vi "WriteCSV.vi"(11 "Log Queue":refnum<queue>) -> (2 "queue out":refnum<queue>, 3 "refnum out":refnum<file>)   [LabVIEW 2026]
uses:
  <vilib>/Platform/TimedLoop/XDataNode/timing_clust.ctl
  <vilib>/Platform/TimedLoop/XDataNode/nitl_modes.ctl
  <vilib>/Platform/TimedLoop/XDataNode/wakeup.ctl
  <vilib>/platform/TimedLoop/XDataNode/XDataNode.xnode
  <vilib>/Platform/TimedLoop/XDataNode/XDNodeRunTimeDep.lvlib
panel:
  in  "datalog":bool
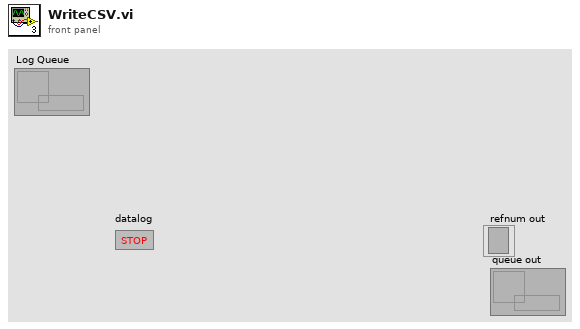
[diagram p1: front panel]
types:
  T1 = enum16{"open", "replace", "create", "open or create", "replace or create", "replace or create with confirmation"}
  T2 = typedef "XDNodeRunTimeDep.lvlib/timing_clust.ctl" = cluster{"Expected End [f-1]":u64, "Actual End [f-1]":u64, "Finished Late? [f-1]":bool, "Expected End [i-1]":u64, "Actual End [i-1]":u64, "Finished Late? [i-1]":bool, "Expected Start [i]":u64, "Actual Start [i]":u64, "Expected Start [f]":u64, "Actual Start [f]":u64, "Source Name":string, "Structure Name":string, "Period":i64, "Deadline":i64, "Offset":i64, "Start":i64, "Priority":i32, "Timeout":i32, "Mode":T3, "Wakeup Reason":T4, "Error":errorcluster, "Source Type":string, "Secondary Source Type":string, "Global End Time":u64, "Global Start Time":u64, "Frame Duration":u64, "Iteration Duration":u64, "Assigned CPU":i32, "I/O Scan Engine Mode":u32}
  T3 = typedef "XDNodeRunTimeDep.lvlib/nitl_modes.ctl" = enum32{"No Change", "Process missed periods, maintain original phase", "Discard missed periods, maintain original phase", "Process missed periods, ignore original phase", "Discard missed periods, ignore original phase"}
  T4 = typedef "XDNodeRunTimeDep.lvlib/wakeup.ctl" = enum32{"Normal", "Aborted", "Asynchronous wakeup", "Timing source error", "Timed loop error", "Timeout"}
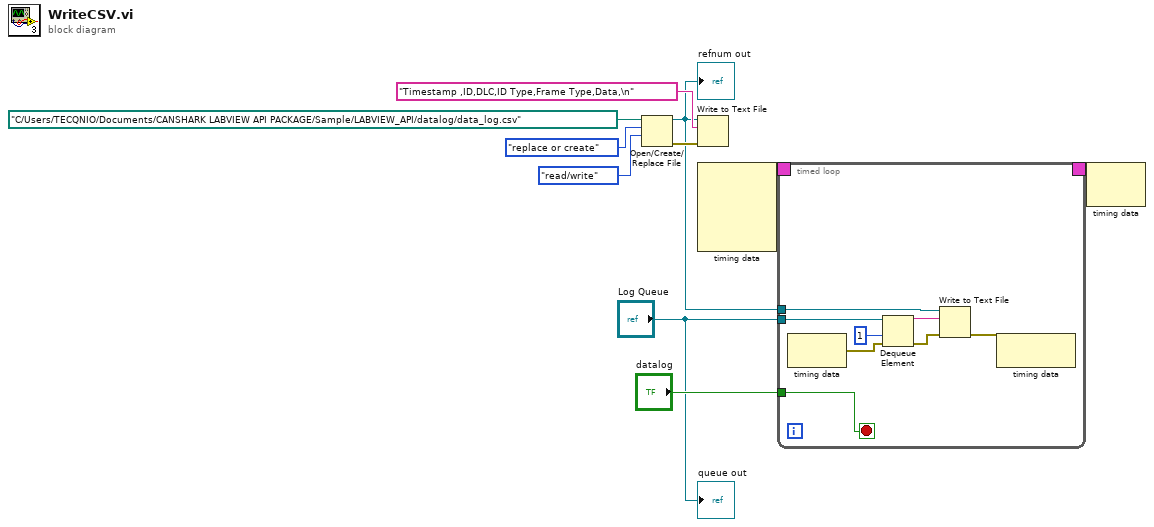
[diagram p0: block diagram]
diagram:
  n1 = Open/Create/Replace File(file path (use dialog)=path "C:/Users/TECQNIO/Documents/CANSHARK LABVIEW API PACKAGE/Sample/LABVIEW_API/datalog/data_log.csv", operation (0:open)=T1."replace or create", access (0:read/write)=enum16{"read/write", "read-only", "write-only"}."read/write") -> (refnum out=w3:refnum<file>, error out=w4:errorcluster)  [unwired: 3 in, 1 out]
  "refnum out" <- w3
  n2 = Write to Text File(file (use dialog)=w3, text="Timestamp ,ID,DLC,ID Type,Frame Type,Data,\n", error in=w4) -> ()  [unwired: 1 in, 3 out]
  n3 = node-c288() -> (w10:T2)  [unwired: 4 in]
  n4 = timed-loop {
    timing: w10 -> [_]
    timing-out: [_] -> w9
    tunnel: "Log Queue" -> [w17]
    tunnel: w3 -> [w15]
    tunnel: "datalog" -> [w14]
    stop <- w14 stop-if-true
    n5 = node-c288() -> (w12:errorcluster)  [unwired: 1 in]
    n6 = Dequeue Element(queue=w17, timeout in ms (-1)=1, error in (no error)=w12) -> (element=w16:string, error out=w11:errorcluster)  [unwired: 2 out]
    n7 = Write to Text File(file (use dialog)=w15, text=w16, error in=w11) -> (error out=w13:errorcluster)  [unwired: 1 in, 2 out]
    n8 = node-c288(w13) -> ()  [unwired: 1 out]
  }
  n9 = node-c288(w9) -> ()  [unwired: 1 out]
  "queue out" <- "Log Queue"
